vi "getFullNodeName.vi"(8 "error in (no error)":errorcluster, 11 "NativeXML in":refnum<class "NativeXML.lvclass">) -> (0 "error out":errorcluster, 2 "fullName":string, 3 "NativeXML out":refnum<class "NativeXML.lvclass">)   [LabVIEW 2011, in "Tools.lvlib" / "xml.lvlib" / "NativeXML.lvclass"]
uses:
  NativeXML.lvclass
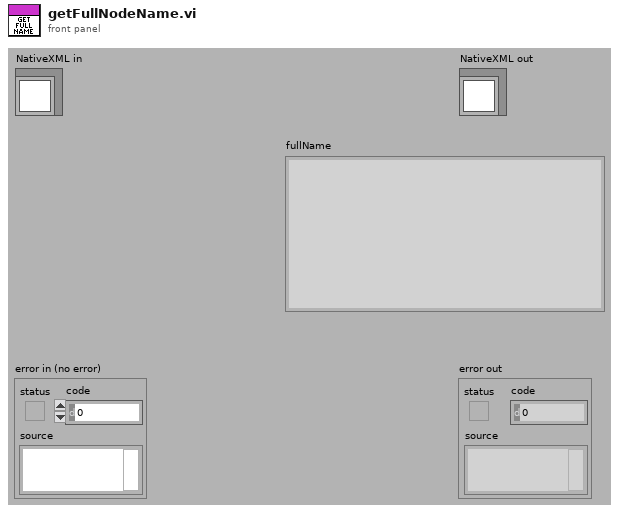
[diagram p1: front panel]
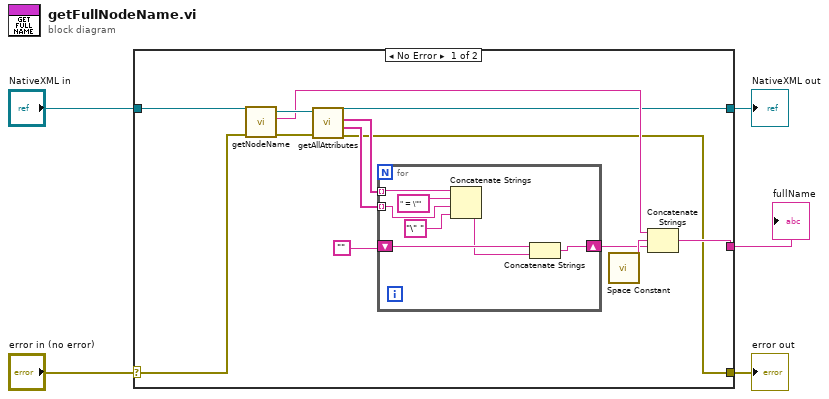
[diagram p0: block diagram]
diagram:
  n1 = case shown="No Error" "error in (no error)" {
    selector: "error in (no error)" -> [w17 w27]
    tunnel: [w6 w27] -> w4
    tunnel: [w7 w26] -> w2
    tunnel: "NativeXML in" -> [w18 w26]
    tunnel: [w8 _] -> w1
    frame No Error {
      n2 = call "getNodeName.vi"("error in (no error)"=w17, "NativeXML in"=w18) -> ("error out"=w15:errorcluster, "name"=w11:string, "NativeXML out"=w16:refnum<class "NativeXML.lvclass">)  [unwired: 7 in]
      n3 = call "getAllAttributes.vi"("error in (no error)"=w15, "NativeXML in"=w16) -> ("error out"=w6:errorcluster, "values"=w13:string[], "names"=w14:string[], "NativeXML out"=w7:refnum<class "NativeXML.lvclass">)  [unwired: 6 in]
      n4 = for {
        tunnel: w14 -> [w25] mode=indexing
        tunnel: w13 -> [w23] mode=indexing
        shift-right: [w21] -> w9
        shift-left: "" -> [w20]
        n5 = Concatenate Strings(w25, " = \"", w23, "\" ") -> (w19:string)
        n6 = Concatenate Strings(w20, w19) -> (w21:string)
      }
      n7 = call <vilib>:"Space Constant.vi"() -> ("String"=w10:string)
      n8 = Concatenate Strings(w11, w10, w9) -> (w8:string)
    }
    frame Error {
    }
  }
  "error out" <- w4
  "NativeXML out" <- w2
  "fullName" <- w1
